vi "Get Gear Ratio.vi"(8 "error in (no error)":errorcluster, 11 "Link In":refnum<class "NI_Robotics_Link.lvclass">) -> (0 "error out":errorcluster, 2 "Gear Ratio":dbl, 3 "Link Out":refnum<class "NI_Robotics_Link.lvclass">)   [LabVIEW 2017, in "NI_Robotics_Link.lvclass"]
uses:
  <vilib>/robotics/Kinematics/Link/NI_Robotics_Link.lvclass
  <vilib>/robotics/Kinematics/Link/NI_Robotics_Link.lvclass/NI_Robotics_Link.ctl
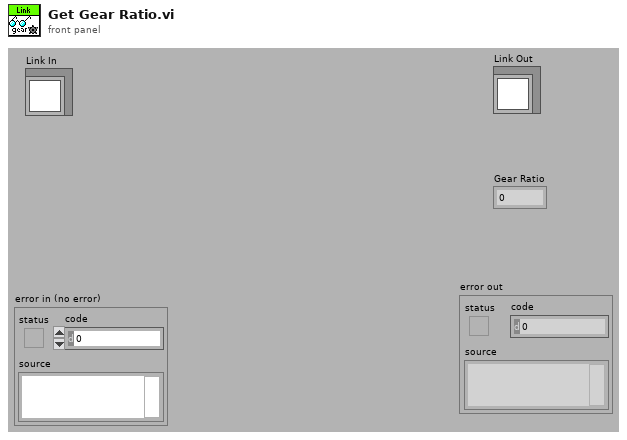
[diagram p1: front panel]
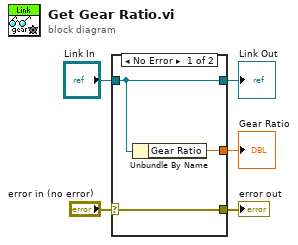
[diagram p0: block diagram]
diagram:
  n1 = case shown="No Error" "error in (no error)" {
    selector: "error in (no error)" -> [w6 w9]
    tunnel: "Link In" -> [w7 w10]
    tunnel: [w8 _] -> w4
    tunnel: [w7 w10] -> w3
    tunnel: [w6 w9] -> w1
    frame No Error {
      n2 = Unbundle By Name(w7) -> ("Gear Ratio"=w8:dbl)
    }
    frame Error {
    }
  }
  "Link Out" <- w3
  "Gear Ratio" <- w4
  "error out" <- w1
